vi "dfd_Coef Report.vi"(8 "error in (no error)":errorcluster, 10 "coefType":u16(ring) items=["b"=7, "a"=0], 11 "filter in":T1={"mSRate_Fs"=1.0, "mSRate_Version"="1.0", "mSRate_Comments"="", "mSRate_OrgCoef"={"type"=enum."Undefined", "gain"=1.0, "coef a (k)"=[], "coef b (v)"=[]}, "mSRate_CurCoef"={"type"=enum."Undefined", "gain"=1.0, "coef a (k)"=[], "coef b (v)"=[]}, "mSRate_Quantized?"=FALSE, "mSRate_QCoef"={"type"=enum."Undefined", "gain"=1.0, "coef a (k)"=[], "coef b (v)"=[]}, "mSRate_QSettings"=[], "mSRate_Order"=0, "mSRate_Scaling"={"mSRate_ScaleByPowerOf2?"=FALSE, "mSRate_ScaleType"=enum."No Norm"}} {"mSRate_QSettings"."source" items=["Coef a/k"=0, "Coef b/v"=7, "Input"=1, "Output"=2, "Multiplicand"=3, "Product"=4, "Sum"=5, "Delay"=6, "Gain"=8]}) -> (0 "error out":errorcluster, 2 "rpt":string, 3 "filter out":T1={"mSRate_Fs"=1.0, "mSRate_Version"="1.0", "mSRate_Comments"="", "mSRate_OrgCoef"={"type"=enum."Undefined", "gain"=1.0, "coef a (k)"=[], "coef b (v)"=[]}, "mSRate_CurCoef"={"type"=enum."Undefined", "gain"=1.0, "coef a (k)"=[], "coef b (v)"=[]}, "mSRate_Quantized?"=FALSE, "mSRate_QCoef"={"type"=enum."Undefined", "gain"=1.0, "coef a (k)"=[], "coef b (v)"=[]}, "mSRate_QSettings"=[], "mSRate_Order"=0, "mSRate_Scaling"={"mSRate_ScaleByPowerOf2?"=FALSE, "mSRate_ScaleType"=enum."No Norm"}} {"mSRate_QSettings"."source" items=["Coef a/k"=0, "Coef b/v"=7, "Input"=1, "Output"=2, "Multiplicand"=3, "Product"=4, "Sum"=5, "Delay"=6, "Gain"=8]})   [LabVIEW 2017, in "NI_DigFilter_FXP.lvlib"]
uses:
  <vilib>/addons/Digital Filter Design/NI_DigFilter_FXP.lvlib
  <vilib>/addons/Digital Filter Design/_Objects.llb/DFD Filter Obj.ctl
  <vilib>/addons/Digital Filter Design/_Objects.llb/DFD Filter Coef.ctl
  <vilib>/addons/Digital Filter Design/_Objects.llb/DFD Filter Structure Type Selector.ctl
  <vilib>/addons/Digital Filter Design/_Objects.llb/dfd_Internal Quantization Settings.ctl
  <vilib>/addons/Digital Filter Design/_Objects.llb/dfd_Internal Quantization Srcs.ctl
  <vilib>/addons/Digital Filter Design/_Objects.llb/DFD Coef Norm Type.ctl
  <vilib>/addons/Digital Filter Design/NI_DigFilterLicensed.lvlib
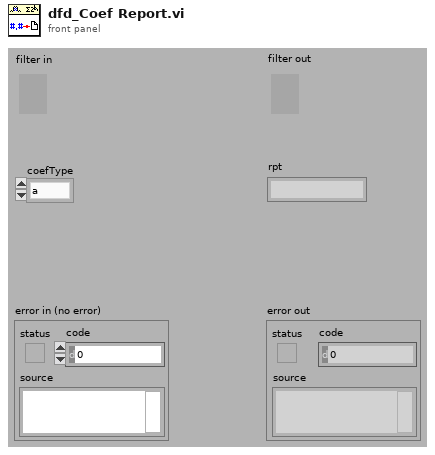
[diagram p1: front panel]
types:
  T1 = typedef "NI_DigFilterLicensed.lvlib/DFD Filter Obj.ctl" = cluster{"mSRate_Fs":dbl, "mSRate_Version":string, "mSRate_Comments":string, "mSRate_OrgCoef":T2, "mSRate_CurCoef":T2, "mSRate_Quantized?":bool, "mSRate_QCoef":T2, "mSRate_QSettings":T4[], "mSRate_Order":i32, "mSRate_Scaling":cluster{"mSRate_ScaleByPowerOf2?":bool, "mSRate_ScaleType":T6}}
  T2 = typedef "NI_DigFilterLicensed.lvlib/DFD Filter Coef.ctl" = cluster{"type":T3, "gain":dbl, "coef a (k)":dbl[], "coef b (v)":dbl[]}
  T3 = typedef "NI_DigFilterLicensed.lvlib/DFD Filter Structure Type Selector.ctl" = enum16{"Undefined", "FIR Direct Form", "FIR Direct Form Transposed", "FIR Symmetric", "FIR Antisymmetric", "IIR Direct Form I", "IIR Direct Form I Transposed", "IIR Direct Form II", "IIR Direct Form II Transposed", "IIR Cascaded Second Order Sections Form I", "IIR Cascaded Second Order Sections Form I Transposed", "IIR Cascaded Second Order Sections Form II", "IIR Cascaded Second Order Sections Form II Transposed", "Lattice Allpass (basic sections)", "Lattice Allpass (one multiplier sections)", "Lattice Allpass (normalized sections)", "Lattice AR (basic sections)", "Lattice AR (one multiplier sections)", "Lattice AR (normalized sections)", "Lattice MA (minimum phase)", "Lattice MA (maximum phase)", "Lattice ARMA (basic sections)", "Lattice ARMA (one multiplier sections)", "Lattice ARMA (normalized sections)"}
  T4 = typedef "NI_DigFilterLicensed.lvlib/dfd_Internal Quantization Settings.ctl" = cluster{"source":T5, "wl":i16, "iwl":i16, "overflow mode":enum16{"Saturation", "Wrap"}, "rounding mode":enum16{"Nearest", "Truncation"}, "signed?":bool}
  T5 = typedef "NI_DigFilterLicensed.lvlib/dfd_Internal Quantization Srcs.ctl" = u16
  T6 = typedef "NI_DigFilterLicensed.lvlib/DFD Coef Norm Type.ctl" = enum16{"No Norm", "Time Domain 1-Norm", "Time Domain 2-Norm", "Time Domain Inf-Norm"}
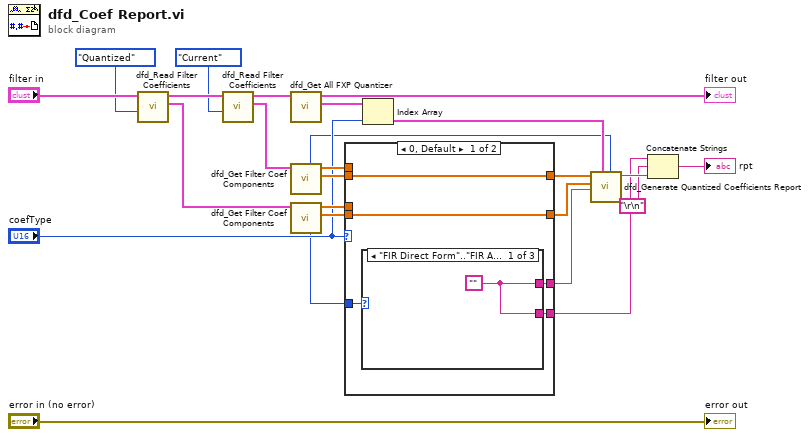
[diagram p0: block diagram]
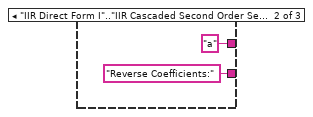
[diagram p2: hidden frame]
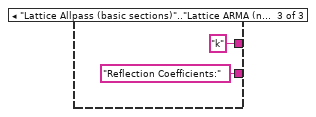
[diagram p3: hidden frame]
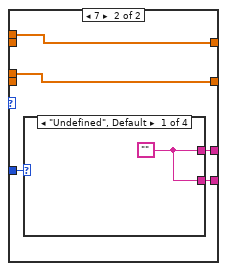
[diagram p4: hidden frame]
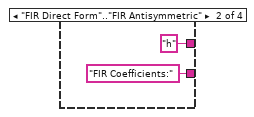
[diagram p5: hidden frame]
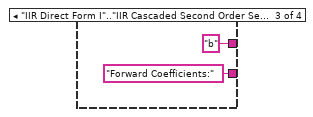
[diagram p6: hidden frame]
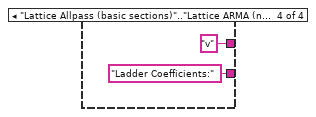
[diagram p7: hidden frame]
diagram:
  n1 = call <vilib>:"dfd_Read Filter Coefficients.vi"("coef source"=enum16{"Original", "Current", "Quantized"}."Quantized", "filter in"="filter in") -> ("filter coef"=w18:T2, "filter out"=w25:T1)  [unwired: 1 in, 7 out]
  n2 = call <vilib>:"dfd_Read Filter Coefficients.vi"("coef source"=enum16{"Original", "Current", "Quantized"}."Current", "filter in"=w25) -> ("filter coef"=w19:T2, "filter out"=w24:T1)  [unwired: 1 in, 7 out]
  n3 = call <vilib>:"dfd_Get All FXP Quantizer.vi"("filter in"=w24) -> ("quantization settings"=w13:T4[], "filter out"=→"filter out":T1)  [unwired: 1 in, 8 out]
  n4 = call <vilib>:"dfd_Get Filter Coef Components.vi"("filter coef"=w19) -> ("coef a (k)"=w16:dbl[], "coef b (v)"=w17:dbl[], "type"=w7:T3)  [unwired: 1 in, 7 out]
  n5 = call <vilib>:"dfd_Get Filter Coef Components.vi"("filter coef"=w18) -> ("coef a (k)"=w14:dbl[], "coef b (v)"=w15:dbl[], "type"=w6:T3)  [unwired: 1 in, 7 out]
  n6 = case shown="0, Default" "coefType" {
    tunnel: w17 -> [_ w40]
    tunnel: w16 -> [w30 _]
    tunnel: w15 -> [_ w39]
    tunnel: w14 -> [w29 _]
    tunnel: [w30 w40] -> w10
    tunnel: [w29 w39] -> w9
    tunnel: w6 -> [w28 w36]
    tunnel: [w27 w38] -> w5
    tunnel: [w26 w37] -> w2
    frame 0, Default {
      n7 = case shown="\"FIR Direct Form\"..\"FIR Antisymmetric\", Default" w28 {
        tunnel: [w31 "a" "k"] -> w27
        tunnel: [w31 "Reverse Coefficients:" "Reflection Coefficients:"] -> w26
        frame "FIR Direct Form".."FIR Antisymmetric", Default {
          w31 = ""
        }
        frame "IIR Direct Form I".."IIR Cascaded Second Order Sections Form II Transposed" {
        }
        frame "Lattice Allpass (basic sections)".."Lattice ARMA (normalized sections)" {
        }
      }
    }
    frame 7 {
      n8 = case shown="\"Undefined\", Default" w36 {
        tunnel: [w41 "h" "b" "v"] -> w38
        tunnel: [w41 "FIR Coefficients:" "Forward Coefficients:" "Ladder Coefficients:"] -> w37
        frame "Undefined", Default {
          w41 = ""
        }
        frame "FIR Direct Form".."FIR Antisymmetric" {
        }
        frame "IIR Direct Form I".."IIR Cascaded Second Order Sections Form II Transposed" {
        }
        frame "Lattice Allpass (basic sections)".."Lattice ARMA (normalized sections)" {
        }
      }
    }
  }
  n9 = Index Array(array=w13, index="coefType") -> (element=w11:T4)
  n10 = call <vilib>:"dfd_Generate Quantized Coefficients Report.vi"("structure type"=w7, "quant settings"=w11, "prefix"=w5, "quantized coef"=w9, "reference coef"=w10) -> ("report"=w4:string)  [unwired: 1 in, 5 out]
  n11 = Concatenate Strings(w2, "\r\n", w4) -> (→"rpt":string)
  "error out" <- "error in (no error)"
